vi "GetBoardByName.vi"(10 "Board Name":string, 11 "Trigger Data":T3) -> (3 "Selected Board":T4)   [LabVIEW 2016]
uses:
  Ctrl_Signal.ctl
  Ctrl_Signal_Map.ctl
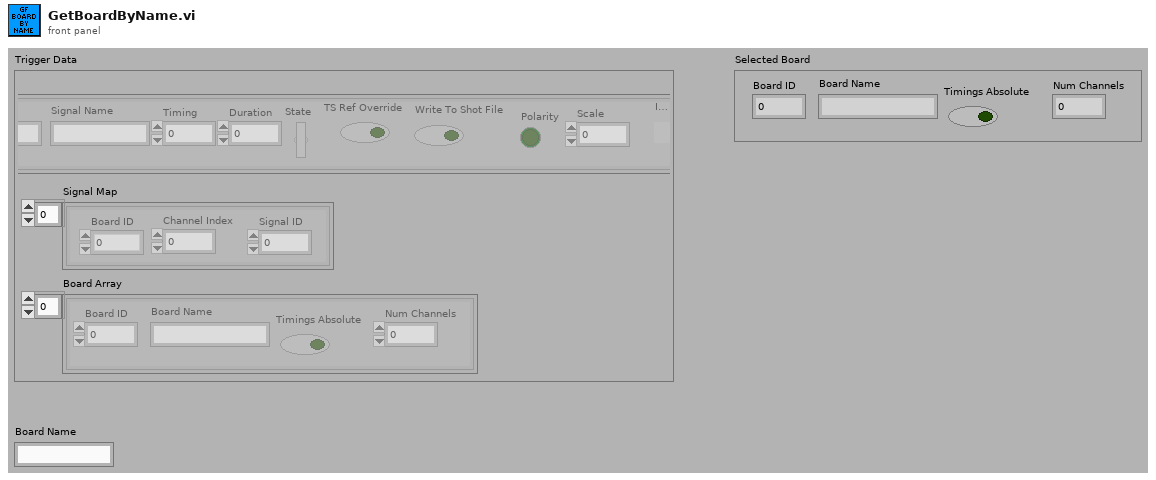
[diagram p1: front panel]
types:
  T1 = typedef "Ctrl_Signal.ctl" = cluster{"Signal Name":string, "Timing":dbl, "Duration":dbl, "State":bool, "TS Ref Override":bool, "Write To Shot File":bool, "Polarity":bool, "Signal ID":dbl, "Scale":dbl, "IsDelay":bool}
  T2 = typedef "Ctrl_Signal_Map.ctl" = cluster{"Channel Index":dbl, "Board ID":dbl, "Signal ID":dbl}
  T3 = cluster{"Signal Array":T1[], "Signal Map":T2[], "Board Array":cluster{"Board ID":dbl, "Board Name":string, "Timings Absolute":bool, "Num Channels":dbl}[]}
  T4 = cluster{"Board ID":dbl, "Board Name":string, "Timings Absolute":bool, "Num Channels":dbl}
  T5 = cluster{"Board ID":dbl, "Board Name":string, "Timings Absolute":bool, "Num Channels":dbl}[]
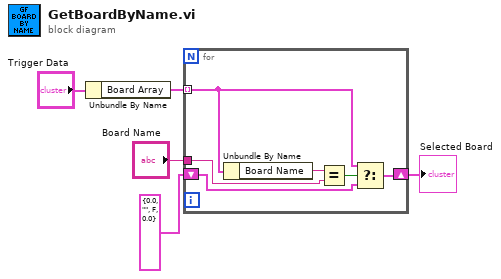
[diagram p0: block diagram]
diagram:
  n1 = Unbundle By Name("Trigger Data") -> ("Board Array"=w1:T5)
  n2 = for {
    tunnel: w1 -> [w6] mode=indexing
    shift-right: [w10] -> w4
    shift-left: T4 {"Board ID"=0.0, "Board Name"="", "Timings Absolute"=FALSE, "Num Channels"=0.0} ("Selected Board") -> [w11]
    tunnel: "Board Name" -> [w8]
    n3 = Unbundle By Name(w6) -> ("Board Name"=w9:string)
    n4 = Equal?(x=w9, y=w8) -> (x = y?=w7:bool)
    n5 = Select(t=w6, s=w7, f=w11) -> (s? t:f=w10:T4)
  }
  "Selected Board" <- w4
